vi "EX_Discrete Swept-Sine Measurements (DAQmx) (Finite).vi"() -> ()   [LabVIEW 2018]
doc: "Overview:\nThis VI demonstrates simultaneous frequency response, level, and distortion measurements using a discrete swept-sine technique. This example implements analog input and analog output with 'Finite Samples' sample mode which minimizes sensitivity to bandwidth issues that can cause run-time errors when performing continuous measurements. This VI also demonstrates how finite acquisitions can be read in a single large block or in a series of smaller reads.\n\nRequirements:\nLabVIEW Full Development System\nSound and Vibration Toolkit\n\nInstructions:\n1. Connect the DUT to the DSA device.\n2. Select the AO excitation channel, AI stimulus channel, and AI response channel.\n3. Run the VI.\n\nDetails:\nThis VI performs a swept sine measurement to obtain the root-mean-square (RMS) levels of the acquired stimulus and response, the frequency response of the device under test (DUT), and the harmonic distortion on the response channel. You specify the source and measurement parameters, and the swept sine VIs handle all the DAQ-specific controls required to perform the measurement. You have direct control over the source, input, averaging, and display parameters. You also specify the engineering units to use for the swept sine measurements.\n\nYou can view the time records of the acquired stimulus and response signals. From these graphs, you can see that the transition to the next test frequency always occurs at a zero crossing to minimize non-linear disturbances to the DUT. The RMS levels, frequency response, and harmonic distortion are shown on different tabs."
uses:
  <vilib>/addons/_NISVFA/_Generation/Signal Generation/SV Signal/SV Signal.lvclass/SV Signal.ctl
  <vilib>/DAQmx/read.llb/DAQmx Read (Analog 1D Wfm NChan NSamp).vi
  <vilib>/addons/Sound and Vibration/svt_Level/SVL AC & DC Level (Time) (1 Ch).vi
  <vilib>/addons/_NISVFA/_Shared subVIs/Common/SV Append Data (N Ch) (DBL).vi
  <vilib>/addons/_NISVFA/_Generation/Signal Generation/SV Signal/Write Leading Synchronization Pulse Enable.vi
  <vilib>/addons/_NISVFA/_Generation/Signal Generation/SV Signal/Read Synchronization Pulse Waveform.vi
  <vilib>/addons/_NISVFA/_Shared subVIs/Common/svc_Get SV Channel Info.vi
  <vilib>/Analysis/baseanly.llb/Mean.vi
  <vilib>/Analysis/baseanly.llb/Mean (DBL).vi
  <vilib>/addons/_NISVFA/_Shared subVIs/Windowing/svfa_Scaled Time Domain Window (Array).vi
  <vilib>/addons/_NISVFA/_Generation/Signal Generation/SV Signal/Read Leading Synchronization Pulse Enable.vi
  <vilib>/addons/_NISVFA/_Generation/Signal Generation/SV Signal/Read Trailing Synchronization Pulse Enable.vi
  <vilib>/Analysis/4window.llb/Force Window.vi
  <vilib>/Analysis/4window.llb/Force Window (DBL).vi
  <vilib>/Analysis/4window.llb/Exponential Window.vi
  <vilib>/Analysis/4window.llb/Exponential Window (DBL).vi
  <vilib>/addons/_NISVFA/_Generation/Signal Generation/SV Discrete Sweep/SV Discrete Sweep.lvclass
  C:/Program Files (x86)/National Instruments/LabVIEW 2018/vi.lib/addons/_NISVFA/_Generation/Signal Generation/SV Signal/SV Signal.lvclass
  C:/Program Files (x86)/National Instruments/LabVIEW 2018/vi.lib/addons/_NISVFA/_Generation/Signal Generation/SV Function/SV Function.lvclass
  <vilib>/DAQmx/create/channels.llb/DAQmx Create Channel (AO-Voltage-Basic).vi
  <vilib>/addons/_NISVFA/_Generation/Signal Generation/SV Discrete Sweep/Configure Frequency Sweep at Constant Amplitude.vi
  <vilib>/DAQmx/create/channels.llb/DAQmx Create Channel (AI-Voltage-Basic).vi
  <vilib>/addons/_NISVFA/_Generation/Signal Generation/SV Signal/Write Ramp Parameters.vi
  <vilib>/addons/_NISVFA/_Generation/Signal Generation/SV Signal/Write DC Offset.vi
  <vilib>/addons/_NISVFA/_Generation/Signal Generation/SV Signal/Write Measurement Duration.vi
  <vilib>/addons/_NISVFA/_Generation/Signal Generation/SV Function/Write Measurement Cycles.vi
  <vilib>/addons/_NISVFA/_Generation/Signal Generation/SV Signal/Write Pre-Measurement Settling Duration.vi
  <vilib>/addons/_NISVFA/_Generation/Signal Generation/SV Function/Write Pre-Measurement Settling Cycles.vi
  <vilib>/addons/_NISVFA/_Generation/Signal Generation/SV Signal/Read System Timing Model.vi
  <vilib>/addons/_NISVFA/_Generation/Signal Generation/SV Signal/Write System Timing Model.vi
  <vilib>/DAQmx/miscellaneous.llb/DAQmx Fill In Error Info.vi
  <vilib>/addons/_NISVFA/_Shared subVIs/Data Objects/Waveforms (DBL)/SV Read Next Measurement Data.vi
  <vilib>/addons/_NISVFA/_Shared subVIs/Common/svc_Get Window Info.vi
  <vilib>/addons/_NISVFA/_Shared subVIs/Common/svc_Unit Label to Engineering Units.vi
  <vilib>/addons/_NISVFA/_Shared subVIs/Common/svc_Engineering Units to Unit Label.vi
  <vilib>/addons/_NISVFA/_Spectrum Processing/subVIs/svfa_Spectrum Info Window to windowTd Type Def.vi
  <vilib>/Analysis/0measdsp.llb/Scaled Time Domain Window.vi
  <vilib>/Analysis/0measdsp.llb/Scaled Time Domain Window (DBL).vi
  <vilib>/Utility/error.llb/Error Cluster From Error Code.vi
  <vilib>/Analysis/baseanly.llb/Std Deviation and Variance.vi
  <vilib>/addons/_NISVFA/_Shared subVIs/Common/svc_Caller VI Returned in Error Source.vi
  <vilib>/addons/Sound and Vibration/svt_Single Tone Measurements/SVT Gain and Phase (Time).vi
  <vilib>/addons/Sound and Vibration/svt_Distortion/SVT THD and Harmonic Components (Frequency) (1 Ch).vi
  <vilib>/addons/_NISVFA/_Generation/Signal Generation/SV Signal/SV Signal.lvclass
  <vilib>/addons/_NISVFA/_Shared subVIs/Data Objects/Waveforms (DBL)/Waveforms (N Ch).lvclass
  <vilib>/addons/Sound and Vibration/svt_Distortion/SoundVib_Distortion.lvlib
  <vilib>/addons/Sound and Vibration/svt_Single Tone Measurements/SoundVib_SingleTone.lvlib
  Program Files (x86)/National Instruments/LabVIEW 2018/examples/Sound and Vibration/SoundVib_Audio Examples.lvlib
  C:/Program Files (x86)/National Instruments/LabVIEW 2018/vi.lib/addons/_NISVFA/_Generation/Signal Generation/SV Sinusoid/SV Sinusoid.lvclass
  <resource>/objmgr/daqmx.rc
panel:
  in  "Read":enum16{"Single", "Multiple"}(ring)=enum."Multiple"
  out "test time":u32
  in  "sweep settings":T1(tab)
  in  "AO source settings":T2={"AO excitation channel"="", "max value [V]"=3.0, "min value [V]"=-3.0, "terminal configuration"=-1} {"terminal configuration" items=["Default"=-1, "RSE"=10083, "Differential"=10106, "Pseudodifferential"=12529]; "min value [V]" format="%0.2f"; "max value [V]" format="%0.2f"}
  in  "AI stimulus settings":T3={"AI stimulus channel"="", "max value [V]"=3.0, "min value [V]"=-3.0, "terminal configuration"=-1} {"terminal configuration" items=["Default"=-1, "RSE"=10083, "NRSE"=10078, "Differential"=10106, "Pseudodifferential"=12529]; "min value [V]" format="%.2f"; "max value [V]" format="%.2f"}
  in  "AI response settings":T4={"AI response channel"="", "max value [V]"=3.0, "min value [V]"=-3.0, "terminal configuration"=-1} {"terminal configuration" items=["Default"=-1, "RSE"=10083, "NRSE"=10078, "Differential"=10106, "Pseudodifferential"=12529]; "min value [V]" format="%.2f"; "max value [V]" format="%.2f"}
  in  "number of steps":i32=190 min=1
  in  "DC offset [V]":dbl format="%.2f"
  in  "amplitude [V]":dbl=1.0 format="%.2p"
  in  "frequency spacing":enum16{"Linear", "Logarithmic"}(ring)=enum."Logarithmic"
  in  "sweep range":cluster{"start":dbl, "stop":dbl}={"start"=20000.0, "stop"=100.0} {"stop" min=0.0 format="%.2f"; "start" min=0.0 format="%.2f"}
  in  "measurement":cluster{"time":dbl, "cycles":dbl}={"time"=0.001, "cycles"=10.0} {"cycles" min=5.0 max=1000.0 step=1.0; "time" min=0.0 max=5.0 step=0.0001 format="%.3f s"}
  in  "settling":cluster{"time":dbl, "cycles":dbl}={"time"=0.0, "cycles"=1.0} {"cycles" min=0.0 max=100.0 step=0.5; "time" min=0.0 max=5.0 step=0.0001 format="%.3f s"}
  out "current frequency":dbl=nan format="%.2f Hz"
  in  "views":T5(tab)
  in  "Getting Started":string="GETTING STARTED\n\nThis VI measures the frequency response of the device under test (DUT) with a swept sine technique. The example generates a discrete frequency sweep for the excitation signal and measures the root-mean-square (RMS) levels of the stimulus and response channels, the frequency response (magnitude and phase), and the total harmonic distortion (THD) (including contributions from individual harmonics) of the DUT. The measurements are performed at each test frequency, one frequency at a time.\n\nRefer to the wiring diagram to physically connect the DSA or DAQ device to the DUT.  This example uses two analog input channels and one analog output channel.  Note that the analog output is connected to both the DUT input and to the first analog input channel on the measurement device.  \n\nThe wiring diagram assumes that you use the default channel settings.  If you change the channel settings in the VI front panel you should adjust the physical connections appropriately.\n\nNI strongly recommends that you take precautions to limit the effects of out-of-band aliasing in your frequency domain measurements.  DSA devices use transparent digital and analog hardware filtering to eliminate aliased input and output frequencies.  Multifunction DAQ devices are more susceptible to the effects of aliased frequencies.  If you are using a non-DSA measurement device, we recommend addressing potential aliasing through high sampling rates, built-in analog filters on S Series devices, and/or external analog filters.\n\nKEY PARAMETERS\n\nDAQ Configuration:AI stimulus channel\n\nThe stimulus channel is the acquired reference. This is the first channel added to the analog input task. Often, this channel will serve as a direct measurement of the excitation channel, but you may also connect after the excitation signal has been conditioned or amplified in order to measure the input to the DUT.\n\nSource Settings:  amplitude [V]\n\nThis control allows you to specify the peak amplitude of the tone used to perform the swept-sine measurement. \n\nSource Settings:  sweep frequencies\n\nThe start frequency and stop frequency determine the frequency range of the swept-sine measurement. You could set the start frequency to be 20 Hz and the stop frequency to be 20 kHz to sweep up in frequency, or you could set the start frequency to be 20 kHz and the stop frequency to be 20 Hz to sweep down in frequency. The number of steps determines the total number of test frequencies.\n\nProcessing Settings: settling\n\nThe \"settle time\" and \"settle cycles\" parameters allow you to specify a delay between the start of the stimulus and the beginning of the measurement.  Some DUTs have a significant transient response to sudden changes in frequency, select the appropriate settling settings to allow this transient response to pass.  At each frequency, the VI will wait for a number of seconds equal to either \"settle time\" or \"settle cycles\" divided by the stimulus frequency, whichever is greater.\n\nProcessing Settings:  measurement\n\nThe \"integration time\" and \"integration cycles\" parameters allow you specify how much data is averaged at each frequency step.  Each average will process data for a number of seconds equal to either \"integration time\" or \"integration cycles\" divided by the stimulus frequency, whichever is greater.\n\nTHD Settings:  maximum harmonic\n\nThis setting determines how many harmonics should contribute to the THD calculation.  For instance, assume the \"maximum harmonic\" is set at 5 and the excitation frequency is set at 2 kHz.  In this case, the THD will be the ratio of the RMS sum of powers at 4 kHz, 6 kHz, 8 kHz, and 10 kHz to the power at 2 kHz (the fundamental).  If you select \"-1\" for this parameter, the VI will compute the power for all harmonics whose frequencies lie below the Nyquist frequency\n\nTHD Settings such as harmonics to visualize and maximum harmonic are set in block-diagram constants."
  out "Response":waveform(dbl)[](graph)
  out "Stimulus":waveform(dbl)[](graph)
  out "RMS level (response)":cluster{"frequency":dbl[], "magnitude":dbl[]}(graph)
  out "RMS level (stimulus)":cluster{"frequency":dbl[], "magnitude":dbl[]}(graph)
  out "Phase":cluster{"frequency":dbl[], "magnitude":dbl[]}(graph)
  out "Magnitude":cluster{"frequency":dbl[], "magnitude":dbl[]}(graph)
  out "Harmonics":cluster{"f":dbl[], "H_i":dbl[]}[](graph)
  out "THD":cluster{"frequency":dbl[], "THD":dbl[]}(graph)
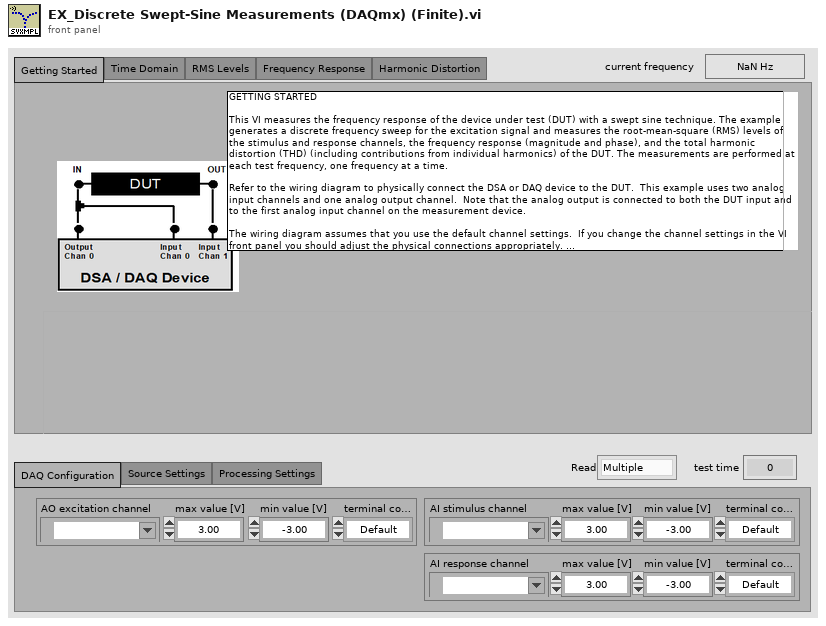
[diagram p1: front panel]
types:
  T1 = enum32{"DAQ Configuration", "Source Settings", "Processing Settings"}
  T2 = cluster{"AO excitation channel":tag, "max value [V]":dbl, "min value [V]":dbl, "terminal configuration":i32}
  T3 = cluster{"AI stimulus channel":tag, "max value [V]":dbl, "min value [V]":dbl, "terminal configuration":i32}
  T4 = cluster{"AI response channel":tag, "max value [V]":dbl, "min value [V]":dbl, "terminal configuration":i32}
  T5 = enum32{"Getting Started", "Time Domain", "RMS Levels", "Frequency Response", "Harmonic Distortion"}
  T6 = cluster{"profile":enum16{"Linear", "Half cosine"}, "durations [s]":cluster{"ramp-up":dbl, "transition":dbl, "ramp-down":dbl}}
  T7 = cluster{"gain units":enum16{"dB", "linear ratio"}, "phase units":enum16{"deg", "rad"}, "detected tone stimulus amplitude units":enum16{"EU rms", "EU peak", "EU peak-peak"}, "detected tone response amplitude units":enum16{"EU rms", "EU peak", "EU peak-peak"}}
  T8 = cluster{"THD units":enum16{"dB", "linear ratio", "%"}, "harmonic component amplitude units":enum16{"EU rms", "EU peak", "EU peak-peak", "dB ref fund"}, "detected fundamental amplitude units":enum16{"EU rms", "EU peak", "EU peak-peak"}}
  T9 = typedef "svc_Spectrum Info.ctl" = cluster{"channel name":string, "description":string, "x-axis units":T10, "spectral info":cluster{"spectrum type":T11, "linear/dB":enum16{"linear", "dB"}, "window":u16, "window size":i32, "FFT size":i32}, "engineering units":T12, "custom label":string, "dB reference [EU]":dbl, "peak units":enum16{"rms", "peak", "peak-peak"}, "weighting filter":T13, "spectral density?":bool, "unit label":string, "spectrum skewed?":bool, "complimentary spectrum units":T14}
  T10 = typedef "svc_X-Axis Units.ctl" = u16
  T11 = typedef "svc_Spectrum Type.ctl" = enum16{"FFT Spectrum [complex]", "Amplitude [Magnitude]", "Power [Magnitude^2]", "Cross Spectrum [complex]", "Frequency Response [Complex]"}
  T12 = typedef "svc_Engineering Units Text Ring.ctl" = u16
  T13 = typedef "svc_Weighting Filter Text Ring.ctl" = u16
  T14 = typedef "svc_Complimentary Spectrum Units.ctl" = enum16{"none", "radians", "degrees", "cycles", "imaginary"}
  T15 = cluster{"complex spectrum response":cluster{"f0":dbl, "df":dbl, "complex spectrum":cdb[]}, "spectrum info":T9}
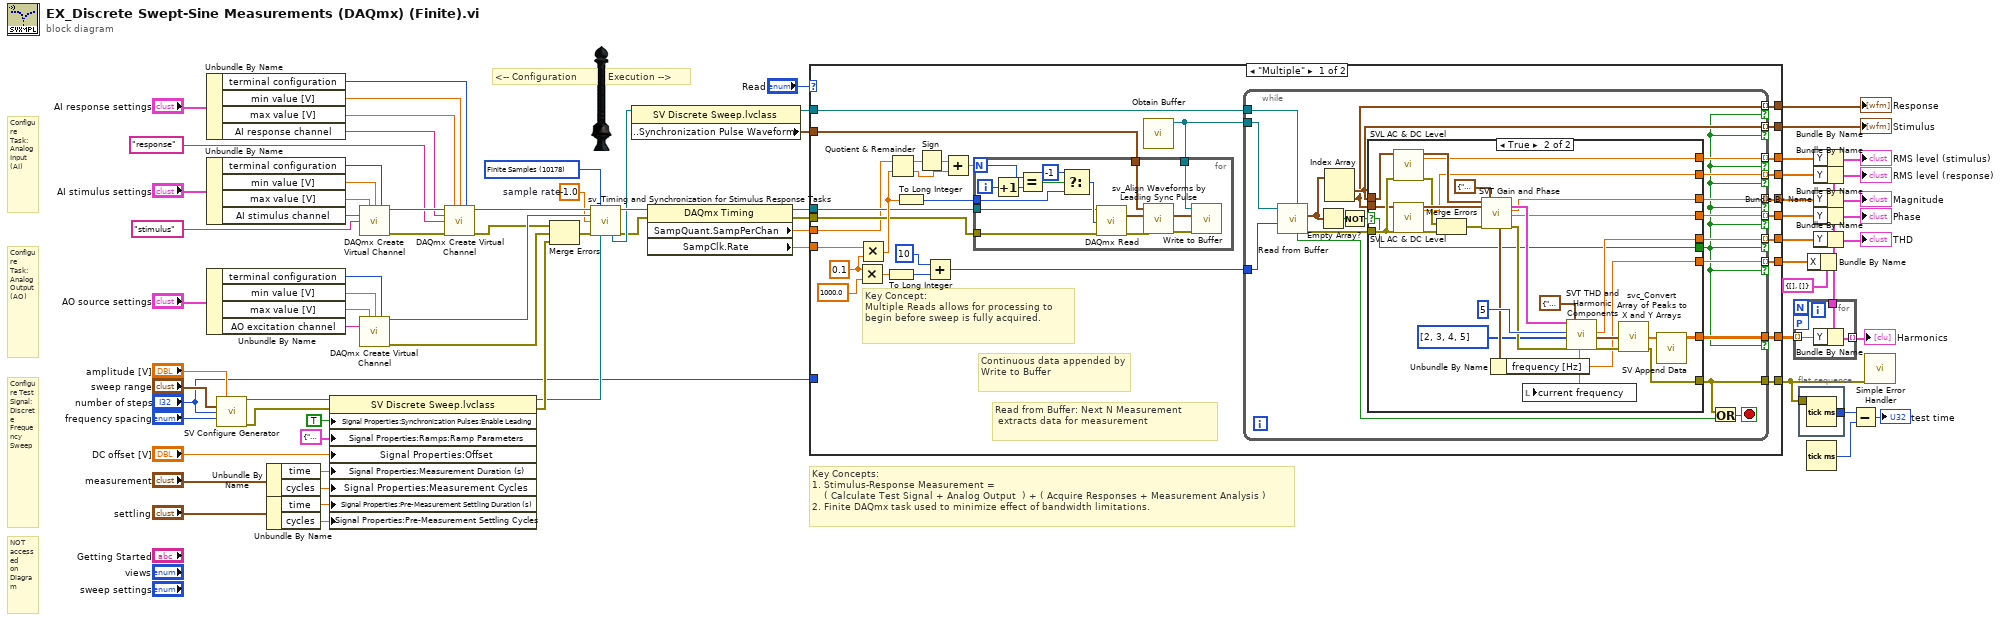
[diagram p0: block diagram]
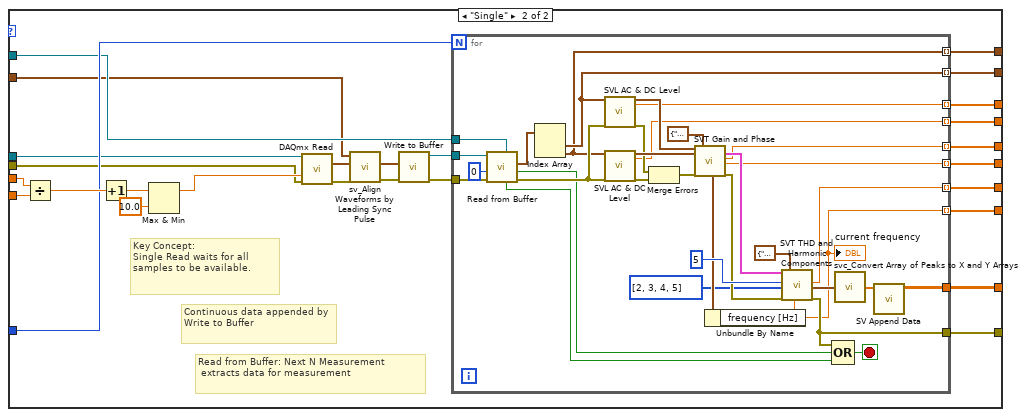
[diagram p3: hidden frame]
diagram:
  w14 = -1.0  # sample rate
  w38 = 10178 items=["Finite Samples"=10178, "Continuous Samples"=10123, "Hardware Timed Single Point"=12522] ("sample mode")
  # "Key Concepts:\n1. Stimulus-Response Measurement = \n    ( Calculate Test Signal + Analog Output  ) + ( Acquire Responses + Measurement Analysis )\n2. Finite DAQmx task used to minimize effect of bandwidth limitations."
  # "NOT accessed\non Diagram"
  # "Execution -->"
  # "<-- Configuration"
  # "Configure Task: \nAnalog Input (AI)"
  # "Configure Task: \nAnalog Output (AO)"
  # "Configure Test Signal: \nDiscrete Frequency Sweep"
  n1 = Unbundle By Name("AI response settings") -> ("terminal configuration"=w56:i32, "min value [V]"=w55:dbl, "max value [V]"=w57:dbl, "AI response channel"=w52:tag)
  n2 = Unbundle By Name("AI stimulus settings") -> ("terminal configuration"=w58:i32, "min value [V]"=w63:dbl, "max value [V]"=w62:dbl, "AI stimulus channel"=w53:tag)
  n3 = Unbundle By Name("AO source settings") -> ("terminal configuration"=w59:i32, "min value [V]"=w60:dbl, "max value [V]"=w61:dbl, "AO excitation channel"=w54:tag)
  n4 = call-poly <vilib>:"SV Configure Generator.vi"("amplitude"="amplitude [V]", "frequency range [Hz]"="sweep range", "number of steps"="number of steps", "profile"="frequency spacing") -> ("signal configuration"=w74:refnum<class "SV Discrete Sweep.lvclass">, "error out"=w44:errorcluster)  [unwired: 10 in]
  n5 = Unbundle By Name("measurement") -> ("time"=w70:dbl, "cycles"=w69:dbl)
  n6 = Unbundle By Name("settling") -> ("time"=w72:dbl, "cycles"=w71:dbl)
  n7 = property class="SV Discrete Sweep.lvclass"(reference=w74, error in=w44, "Signal Properties:Synchronization Pulses:Enable Leading"=TRUE ("Synchronization Pulses:Enable Leading"), "Signal Properties:Ramps:Ramp Parameters"=T6 {"profile"=enum."Half cosine", "durations [s]"={"ramp-up"=0.01, "transition"=0.0, "ramp-down"=0.01}} ("Ramp Parameters"), "Signal Properties:Offset"="DC offset [V]", "Signal Properties:Measurement Duration (s)"=w70, "Signal Properties:Measurement Cycles"=w69, "Signal Properties:Pre-Measurement Settling Duration (s)"=w72, "Signal Properties:Pre-Measurement Settling Cycles"=w71) -> (reference out=w34:refnum<class "SV Discrete Sweep.lvclass">, error out=w36:errorcluster)
  n8 = call-poly <vilib>:"DAQmx Create Virtual Channel.vi"("maximum value"=w62, "minimum value"=w63, "input terminal configuration"=w58, "physical channels"=w53, "name to assign"="stimulus") -> ("task out"=w65:refnum<k21>, "error out"=w64:errorcluster)  [unwired: 9 in]
  n9 = call-poly <vilib>:"DAQmx Create Virtual Channel.vi"("maximum value"=w61, "minimum value"=w60, "output terminal configuration"=w59, "physical channels"=w54) -> ("task out"=w42:refnum<k21>, "error out"=w40:errorcluster)  [unwired: 10 in]
  n10 = call-poly <vilib>:"DAQmx Create Virtual Channel.vi"("task in"=w65, "maximum value"=w57, "minimum value"=w55, "input terminal configuration"=w56, "physical channels"=w52, "name to assign"="response", "error in"=w64) -> ("task out"=w43:refnum<k21>, "error out"=w41:errorcluster)  [unwired: 7 in]
  n11 = Merge Errors(w41, w40, w36) -> (w39:errorcluster)
  n12 = call "sv_Timing and Synchronization for Stimulus Response Tasks.vi"("analog input task"=w43, "sample mode"=w38, "analog output task"=w42, "sample rate (Hz)"=w14, "error in (no error)"=w39, "signal configuration in"=w34) -> ("analog input task"=w37:refnum<k21>, "signal configuration out"=w30:refnum<class "SV Discrete Sweep.lvclass">, "error out"=w1:errorcluster)  [unwired: 4 in, 3 out]
  n13 = property class="SV Discrete Sweep.lvclass"(reference=w30) -> (reference out=w33:refnum<class "SV Discrete Sweep.lvclass">, "Signal Properties:Synchronization Pulses:Synchronization Pulse Waveform"=w32:waveform(dbl))  [unwired: 1 in, 1 out]
  n14 = property class="DAQmx Timing"(reference=w37, error in=w1) -> (reference out=w5:refnum<k21>, error out=w4:errorcluster, "SampQuant.SampPerChan"=w3:dbl, "SampClk.Rate"=w2:dbl)
  n15 = case shown="\"Multiple\"" "Read" {
    tunnel: w33 -> [w103 w172]
    tunnel: w32 -> [w102 w171]
    tunnel: [w101 w188] -> w10
    tunnel: "number of steps" -> [_ w182]
    tunnel: [w100 w181] -> w24
    tunnel: [w99 w180] -> w23
    tunnel: [w98 w179] -> w22
    tunnel: [w97 w178] -> w21
    tunnel: [w96 w177] -> w20
    tunnel: [w95 w176] -> w16
    tunnel: [w94 w175] -> w15
    tunnel: [w93 w174] -> w13
    tunnel: [w92 w173] -> w12
    tunnel: w5 -> [w78 w170]
    tunnel: w4 -> [w77 w169]
    tunnel: w3 -> [w76 w168]
    tunnel: w2 -> [w75 w167]
    frame "Multiple" {
      w88 = 0.1 ("read duration")
      # "Key Concept:\nMultiple Reads allows for processing to begin before sweep is fully acquired."
      # "Read from Buffer: Next N Measurement\n extracts data for measurement"
      # "Continuous data appended by Write to Buffer"
      n16 = Multiply(x=w88, y=1000.0) -> (x*y=w84:dbl)
      n17 = Multiply(x=w75, y=w88) -> (x*y=w83:dbl)
      n18 = To Long Integer(number=w84) -> (32bit integer=w80:i32)
      n19 = Quotient & Remainder(x=w76, y=w83) -> (x-y*floor(x/y)=w91:dbl, floor(x/y)=w89:dbl)
      n20 = To Long Integer(number=w83) -> (32bit integer=w82:i32)
      n21 = Sign(1:w91) -> (0:w90:dbl)
      n22 = Add(x=10 ("y"), y=w80) -> (x+y=w79:i32)
      n23 = Add(x=w90, y=w89) -> (x+y=w85:dbl)
      n24 = call <vilib>:"Obtain Buffer.vi"() -> ("buffer out"=w87:refnum<data-value>)  [unwired: 10 in, 1 out]
      n25 = for {
        N: w85 -> [w109]
        tunnel: w102 -> [w118]
        tunnel: w87 -> [w113]
        tunnel: w82 -> [w112]
        tunnel: w78 -> [w105]
        tunnel: w77 -> [w104]
        i -> [w110]
        n26 = Increment(x=w110) -> (x+1=w111:i32)
        n27 = Equal?(x=w109, y=w111) -> (x = y?=w108:bool)
        n28 = Select(t=-1 ("f"), s=w108, f=w112) -> (s? t:f=w106:i32)
        n29 = call-poly <vilib>:"DAQmx Read.vi"("task/channels in"=w105, "number of samples per channel"=w106, "error in"=w104) -> ("data"=w115:waveform(dbl)[], "error out"=w114:errorcluster)  [unwired: 10 in, 1 out]
        n30 = call "sv_Align Waveforms by Leading Sync Pulse.vi"("error in (no error)"=w114, "response signals"=w115, "alignment reference signal"=w118) -> ("error out"=w117:errorcluster, "aligned signals"=w116:waveform(dbl)[])  [unwired: 4 in, 3 out]
        n31 = call <vilib>:"Write to Buffer.vi"("error in (no error)"=w117, "waveforms"=w116, "buffer"=w113) -> ()  [unwired: 6 in, 3 out]
      }
      n32 = while {
        tunnel: w87 -> [w136]
        tunnel: w103 -> [w135]
        tunnel: [w119] -> w101
        tunnel: [w134] -> w100 mode=indexing if=w122
        tunnel: [w133] -> w99 mode=indexing if=w122
        tunnel: [w132] -> w98 mode=indexing if=w122
        tunnel: [w131] -> w97 mode=indexing if=w122
        tunnel: [w130] -> w96 mode=indexing if=w122
        tunnel: [w126] -> w95 mode=indexing if=w122
        tunnel: [w129] -> w94 if=w122
        tunnel: [w128] -> w93 mode=indexing if=w122
        tunnel: [w127] -> w92 mode=indexing if=w122
        tunnel: w79 -> [w121]
        stop <- w125 stop-if-true
        n33 = call-poly <vilib>:"Read from Buffer.vi"("test signal configuration"=w135, "timeout (1000 ms)"=w121, "buffer"=w136) -> ("error out"=w138:errorcluster, "waveforms subset"=w124:waveform(dbl)[], "done"=w137:bool)  [unwired: 4 in, 2 out]
        n34 = Empty Array?(array=w124) -> (empty?=w123:bool)
        n35 = Index Array(array=w124) -> (element #1=w128:waveform(dbl), element #2=w127:waveform(dbl))  [unwired: 2 in]
        n36 = Not(x=w123) -> (.not. x?=w120:bool)
        n37 = case shown="True" w120 {
          selector: w120 -> [w140 w142]
          tunnel: w138 -> [w139 w166]
          tunnel: [w139 w165] -> w119
          tunnel: [_ w151] -> w134
          tunnel: [_ w150] -> w133
          tunnel: [_ w149] -> w132
          tunnel: [_ w148] -> w131
          tunnel: [_ w147] -> w130
          tunnel: [_ w145] -> w129
          tunnel: w128 -> [_ w144]
          tunnel: w127 -> [_ w143]
          tunnel: [_ w141] -> w126
          tunnel: [w140 w142] -> w122
          frame False {
          }
          frame True {
            n38 = call-poly <vilib>:"SVL AC & DC Level.vi"("scaled signal [EU]"=w144, "error in (no error)"=w166) -> ("AC signal [EU]"=w159:waveform(dbl), "AC level [EU rms]"=w151:dbl, "error out"=w156:errorcluster)  [unwired: 12 in, 3 out]
            n39 = call-poly <vilib>:"SVL AC & DC Level.vi"("scaled signal [EU]"=w143, "error in (no error)"=w166) -> ("AC signal [EU]"=w158:waveform(dbl), "AC level [EU rms]"=w150:dbl, "error out"=w155:errorcluster)  [unwired: 12 in, 3 out]
            n40 = Merge Errors(w156, w155) -> (w154:errorcluster)
            n41 = call-poly <vilib>:"SVT Gain and Phase.vi"("stimulus signal X [EUx]"=w159, "response signal Y [EUy]"=w158, "error in (no error)"=w154, "desired units"=T7 {"gain units"=enum."dB", "phase units"=enum."deg", "detected tone stimulus amplitude units"=enum."EU rms", "detected tone response amplitude units"=enum."EU rms"}) -> ("detected tone response"=w153:cluster{"frequency [Hz]":dbl, "amplitude":dbl}, "complex spectrum\nresponse Y"=w160:T15, "gain"=w149:dbl, "phase lag"=w148:dbl, "error out"=w157:errorcluster)  [unwired: 8 in, 3 out]
            n42 = Unbundle By Name(w153) -> ("frequency [Hz]"=w141:dbl)
            n43 = local write "current frequency"(w141) -> ()
            n44 = call-poly <vilib>:"SVT THD and Harmonic Components.vi"("complex spectrum"=w160, "maximum harmonic"=5, "harmonics to visualize"=i32[] [2, 3, 4, 5], "error in (no error)"=w157, "desired units"=T8 {"THD units"=enum."dB", "harmonic component amplitude units"=enum."dB ref fund", "detected fundamental amplitude units"=enum."EU peak"}, "expected fundamental frequency [Hz]"=w141) -> ("THD"=w147:dbl, "harmonic components"=w161:cluster{"frequency [Hz]":dbl, "amplitude":dbl}[], "error out"=w165:errorcluster)  [unwired: 6 in, 5 out]
            n45 = call <vilib>:"svc_Convert Array of Peaks to X and Y Arrays.vi"("peaks"=w161) -> ("Y"=w146:dbl[])  [unwired: 3 in, 1 out]
            n46 = call-poly <vilib>:"SV Append Data.vi"("data in"=w146) -> ("appended data"=w145:dbl[][])  [unwired: 10 in]
          }
        }
        n47 = Or(x=w119, y=w137) -> (x .or. y?=w125:bool)
      }
    }
    frame "Single" {
      # "Read from Buffer: Next N Measurement\n extracts data for measurement"
      # "Continuous data appended by Write to Buffer"
      # "Key Concept:\nSingle Read waits for all samples to be available."
      n48 = Divide(x=w168, y=w167) -> (x/y=w186:dbl)
      n49 = Increment(x=w186) -> (x+1=w185:dbl)
      n50 = Max & Min(x=w185, y=10.0) -> (max(x,y)=w183:dbl)  [unwired: 1 out]
      n51 = call-poly <vilib>:"DAQmx Read.vi"("task/channels in"=w170, "timeout"=w183, "error in"=w169) -> ("data"=w189:waveform(dbl)[], "error out"=w187:errorcluster)  [unwired: 10 in, 1 out]
      n52 = call "sv_Align Waveforms by Leading Sync Pulse.vi"("error in (no error)"=w187, "response signals"=w189, "alignment reference signal"=w171) -> ("error out"=w191:errorcluster, "aligned signals"=w190:waveform(dbl)[])  [unwired: 4 in, 3 out]
      n53 = call <vilib>:"Write to Buffer.vi"("error in (no error)"=w191, "waveforms"=w190) -> ("error out"=w192:errorcluster, "buffer out"=w193:refnum<data-value>)  [unwired: 7 in, 1 out]
      n54 = for {
        N: w182 -> [_]
        tunnel: w193 -> [w223]
        tunnel: w172 -> [w222]
        tunnel: w192 -> [w221]
        tunnel: [w218] -> w188
        tunnel: [w203] -> w181 mode=indexing
        tunnel: [w202] -> w180 mode=indexing
        tunnel: [w201] -> w179 mode=indexing
        tunnel: [w200] -> w178 mode=indexing
        tunnel: [w199] -> w177 mode=indexing
        tunnel: [w198] -> w176 mode=indexing
        tunnel: [w196] -> w175
        tunnel: [w195] -> w174 mode=indexing
        tunnel: [w194] -> w173 mode=indexing
        stop <- w217 stop-if-true
        n55 = call-poly <vilib>:"Read from Buffer.vi"("test signal configuration"=w222, "error in (no error)"=w221, "timeout (1000 ms)"=0, "buffer"=w223) -> ("error out"=w226:errorcluster, "end of buffer"=w219:bool, "waveforms subset"=w220:waveform(dbl)[], "done"=w225:bool)  [unwired: 3 in, 1 out]
        n56 = Index Array(array=w220) -> (element #1=w195:waveform(dbl), element #2=w194:waveform(dbl))  [unwired: 2 in]
        n57 = call-poly <vilib>:"SVL AC & DC Level.vi"("scaled signal [EU]"=w195, "error in (no error)"=w226) -> ("AC signal [EU]"=w211:waveform(dbl), "AC level [EU rms]"=w203:dbl, "error out"=w208:errorcluster)  [unwired: 12 in, 3 out]
        n58 = call-poly <vilib>:"SVL AC & DC Level.vi"("scaled signal [EU]"=w194, "error in (no error)"=w226) -> ("AC signal [EU]"=w210:waveform(dbl), "AC level [EU rms]"=w202:dbl, "error out"=w207:errorcluster)  [unwired: 12 in, 3 out]
        n59 = Merge Errors(w208, w207) -> (w206:errorcluster)
        n60 = call-poly <vilib>:"SVT Gain and Phase.vi"("stimulus signal X [EUx]"=w211, "response signal Y [EUy]"=w210, "error in (no error)"=w206, "desired units"=T7 {"gain units"=enum."dB", "phase units"=enum."deg", "detected tone stimulus amplitude units"=enum."EU rms", "detected tone response amplitude units"=enum."EU rms"}) -> ("detected tone response"=w205:cluster{"frequency [Hz]":dbl, "amplitude":dbl}, "complex spectrum\nresponse Y"=w212:T15, "gain"=w201:dbl, "phase lag"=w200:dbl, "error out"=w209:errorcluster)  [unwired: 8 in, 3 out]
        n61 = Unbundle By Name(w205) -> ("frequency [Hz]"=w198:dbl)
        "current frequency" <- w198
        n62 = call-poly <vilib>:"SVT THD and Harmonic Components.vi"("complex spectrum"=w212, "maximum harmonic"=5, "harmonics to visualize"=i32[] [2, 3, 4, 5], "error in (no error)"=w209, "desired units"=T8 {"THD units"=enum."dB", "harmonic component amplitude units"=enum."dB ref fund", "detected fundamental amplitude units"=enum."EU peak"}, "expected fundamental frequency [Hz]"=w198) -> ("THD"=w199:dbl, "harmonic components"=w213:cluster{"frequency [Hz]":dbl, "amplitude":dbl}[], "error out"=w218:errorcluster)  [unwired: 6 in, 5 out]
        n63 = Compound Arithmetic op=OR(w218, w219, w225) -> (w217:bool)
        n64 = call <vilib>:"svc_Convert Array of Peaks to X and Y Arrays.vi"("peaks"=w213) -> ("Y"=w197:dbl[])  [unwired: 3 in, 1 out]
        n65 = call-poly <vilib>:"SV Append Data.vi"("data in"=w197) -> ("appended data"=w196:dbl[][])  [unwired: 10 in]
      }
    }
  }
  "Stimulus" <- w13
  "Response" <- w12
  n66 = flat-sequence {
    tunnel: w10 -> [_]
    tunnel: [w227] -> w9
    frame #0 {
      n67 = Tick Count (ms)() -> (millisecond timer value=w227:u32)
    }
  }
  n68 = Tick Count (ms)() -> (millisecond timer value=w7:u32)
  n69 = Bundle By Name(cluster=cluster{"X":dbl[], "Y":dbl[]} {"X"=[], "Y"=[]} ("THD vs Amplitude"), "X"=w16) -> (w17:cluster{"X":dbl[], "Y":dbl[]})
  n70 = for {
    tunnel: [w230] -> w19 mode=indexing
    tunnel: w17 -> [w229]
    workers-P: _ -> [_]
    tunnel: w15 -> [w228] mode=indexing
    n71 = Bundle By Name(cluster=w229, "Y"=w228) -> (w230:cluster{"X":dbl[], "Y":dbl[]})
  }
  "Harmonics" <- w19
  n72 = Bundle By Name(cluster=w17, "Y"=w24) -> (→"RMS level (stimulus)":cluster{"X":dbl[], "Y":dbl[]})
  n73 = Bundle By Name(cluster=w17, "Y"=w23) -> (→"RMS level (response)":cluster{"X":dbl[], "Y":dbl[]})
  n74 = Bundle By Name(cluster=w17, "Y"=w22) -> (→"Magnitude":cluster{"X":dbl[], "Y":dbl[]})
  n75 = Bundle By Name(cluster=w17, "Y"=w21) -> (→"Phase":cluster{"X":dbl[], "Y":dbl[]})
  n76 = Bundle By Name(cluster=w17, "Y"=w20) -> (→"THD":cluster{"X":dbl[], "Y":dbl[]})
  n77 = Subtract(x=w9, y=w7) -> (x-y=→"test time":u32)
  n78 = call <vilib>:"Simple Error Handler.vi"("error in (no error)"=w10) -> ()  [unwired: 4 in, 5 out]
